vi "Lab4_main.vi"() -> ()   [LabVIEW 2022 SP3]
panel:
  in  "PD Gain":cluster{"Kd":dbl, "Kp":dbl}={"Kd"=0.58, "Kp"=27.94}
  out "Error Simulation Vs Actaual":cluster{"V":dbl, "Vm (V)":dbl}(graph)
  out "Input V Simulation vs Actual":cluster{"V":dbl, "Vm (V)":dbl}(graph)
  in  "System Parameters":cluster{"a1":dbl, "a0":dbl, "a2 ":dbl, "b":dbl}={"a1"=0.0729, "a0"=0.0, "a2 "=0.002, "b"=0.1282}
  out "Theta Simulation vs Actual":T1(graph)
  in  "Ring":u16(ring) items=["square", "triangle", "sinusoidal"]
  in  "Frequency":dbl=0.8
  in  "Amplitude":dbl=1.0
  in  "dt (s)":dbl=0.01
  in  "On/Off":bool
  out "?":bool
  in  "stop":bool
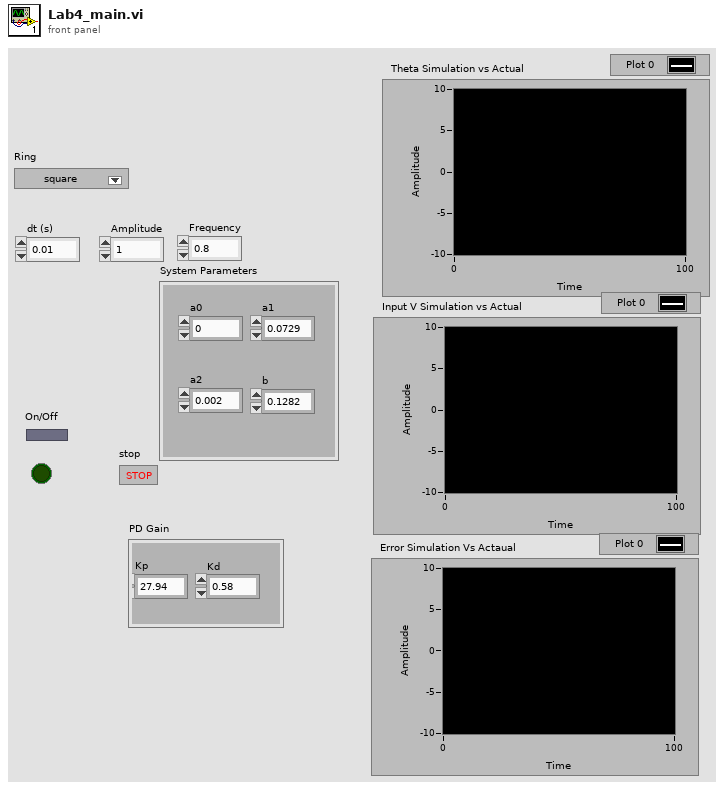
[diagram p1: front panel]
types:
  T1 = cluster{"Theta Out":dbl, "Signal Gen":dbl, "position (rad)":dbl}
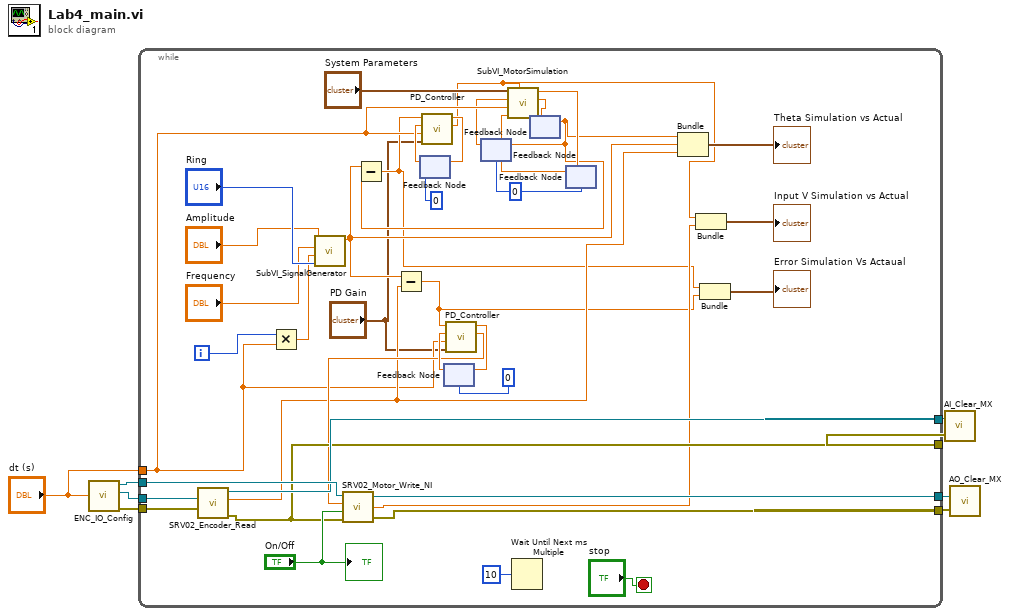
[diagram p0: block diagram]
diagram:
  n1 = call "ENC_IO_Config.vi"("dt"="dt (s)") -> ("AO Task"=w3:refnum<k21>, "ENC Task"=w4:refnum<k21>, "IO error out"=w5:errorcluster)  [unwired: 2 in, 1 out]
  n2 = while {
    tunnel: [w45] -> w8
    tunnel: [w44] -> w7
    tunnel: "dt (s)" -> [w24]
    tunnel: w5 -> [w38]
    tunnel: w4 -> [w37]
    tunnel: w3 -> [w36]
    tunnel: [w35] -> w2
    tunnel: [w34] -> w1
    i -> [w43]
    stop <- "stop" stop-if-true
    w20 = 0
    n3 = call "SRV02_Encoder_Read.vi"("task/channels in"=w37, "error in"=w38) -> ("task out"=w35:refnum<k21>, "position (rad)"=w29:dbl, "error out"=w34:errorcluster)  [unwired: 1 out]
    n4 = Multiply(x=w43, y=w24) -> (x*y=w39:dbl)
    n5 = call "SubVI_SignalGenerator.vi"("Signal Type"="Ring", "Time"=w39, "Freq"="Frequency", "Amplitude"="Amplitude") -> ("Signal Gen"=w19:dbl)  [unwired: 7 in]
    n6 = Subtract(x=w19, y=w29) -> (x-y=w11:dbl)
    n7 = feedback #1(0) -> (w27:dbl)
    n8 = feedback #2(0) -> (w32:dbl)
    n9 = call "PD_Controller.vi"("PD Gain"="PD Gain", "dt"=w24, "Error (n-1)"=w32, "Error"=w11) -> ("V"=w30:dbl, "Error Out"=w33:dbl)  [unwired: 6 in]
    n10 = call "SRV02_Motor_Write_NI.vi"("error in"=w34, "operate?"="On/Off", "u (V)"=w30, "task in"=w36) -> ("error out"=w44:errorcluster, "Vm (V)"=w15:dbl, "task out"=w45:refnum<k21>)
    n11 = feedback-in #2(w33) -> ()
    n12 = feedback #3(w20) -> (w23:dbl)
    n13 = Wait Until Next ms Multiple(millisecond multiple=10) -> ()  [unwired: 1 out]
    n14 = feedback #4() -> (w16:dbl)  [unwired: 1 in]
    n15 = Subtract(x=w19, y=w16) -> (x-y=w10:dbl)
    n16 = call "PD_Controller.vi"("PD Gain"="PD Gain", "dt"=w24, "Error (n-1)"=w27, "Error"=w10) -> ("V"=w13:dbl, "Error Out"=w28:dbl)  [unwired: 6 in]
    n17 = feedback-in #1(w28) -> ()
    n18 = feedback-in #3(w16) -> ()
    n19 = feedback #5(w20) -> (w21:dbl)
    n20 = call "SubVI_MotorSimulation.vi"("Input Voltage"=w13, "Velocity Reading"=w21, "dt [s]"=w24, "Position Reading"=w23, "System Parameters"="System Parameters") -> ("Theta Out"=w17:dbl, "Thetadot Out"=w22:dbl)  [unwired: 5 in]
    n21 = feedback-in #4(w17) -> ()
    n22 = feedback-in #5(w22) -> ()
    n23 = Bundle("Theta Out"=w16, "Signal Gen"=w19, "position (rad)"=w29) -> (→"Theta Simulation vs Actual":T1)  [unwired: 1 in]
    n24 = Bundle("V"=w13, "Vm (V)"=w15) -> (→"Input V Simulation vs Actual":cluster{"V":dbl, "Vm (V)":dbl})  [unwired: 1 in]
    n25 = Bundle(w10, w11) -> (→"Error Simulation Vs Actaual":cluster{dbl, dbl})  [unwired: 1 in]
    "?" <- "On/Off"
  }
  n26 = call "AI_Clear_MX.vi"("Error in"=w1, "Task in"=w2) -> ()  [unwired: 1 out]
  n27 = call "AO_Clear_MX.vi"("Error in"=w7, "Task in"=w8) -> ()  [unwired: 1 out]
